vi "OtherDataType.vi"() -> ()   [LabVIEW 2023]
panel:
  out "data":dbl
  out "variant":variant
  in  "Numeric":dbl
  out "Text Ring 2":u16(ring) items=["동", "서", "남", "북"]
  in  "Text Ring":u16(ring) items=["동", "서", "남", "북"]
  out "Array":dbl[](array[numeric])
  out "Sine":dynamicdata(graph)
  out "Waveform Chart":T1(graph)
  in  "stop 3":bool
  out "Waveform Graph 2":dbl[][](graph)
  in  "stop 2":bool
  in  "stop":bool
  out "Waveform Graph":cluster{dbl, dbl, dbl[]}(graph)
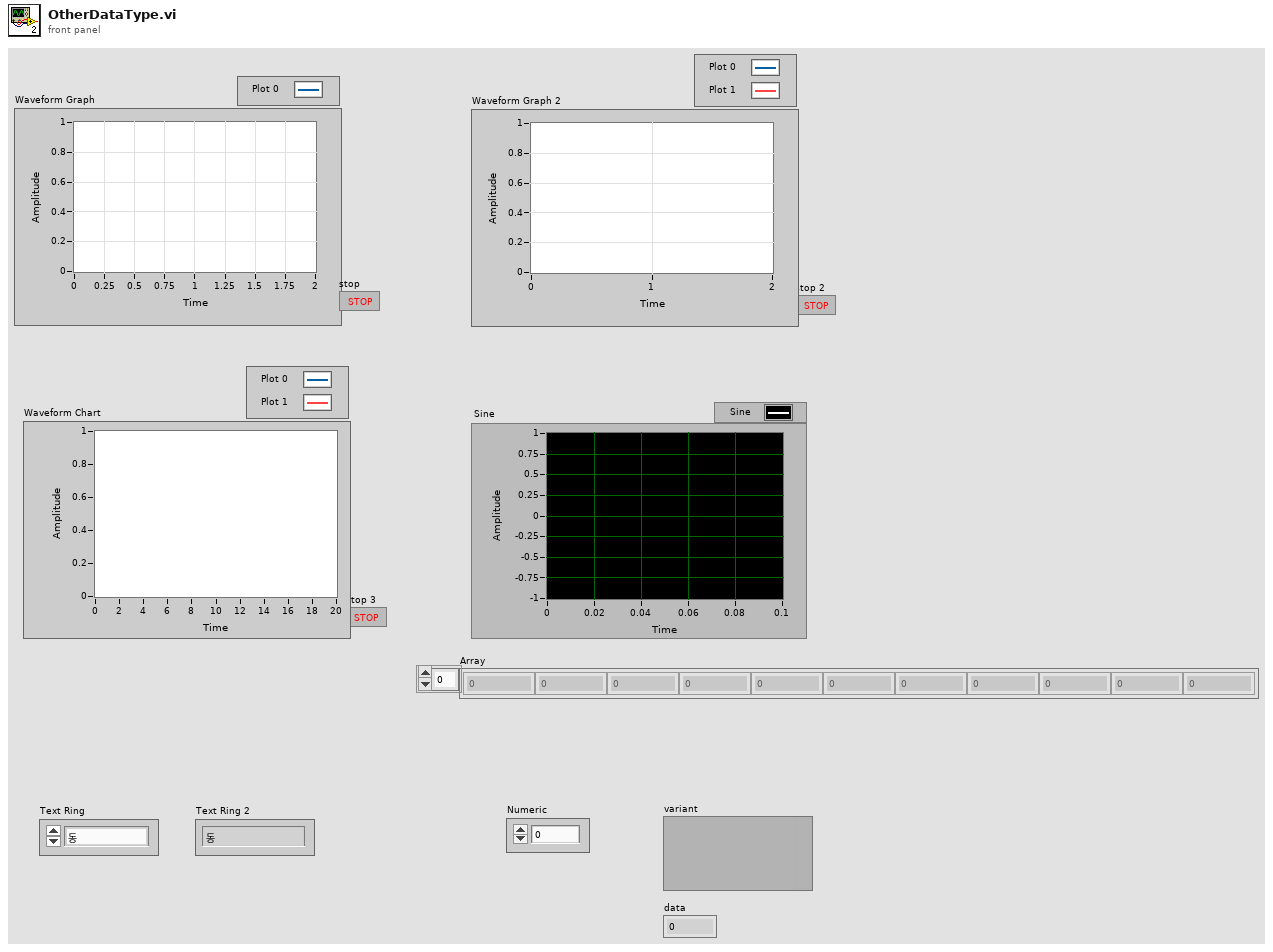
[diagram p1: front panel]
types:
  T1 = cluster{"number: 0 to 1":dbl, "number: 0 to 1":dbl}
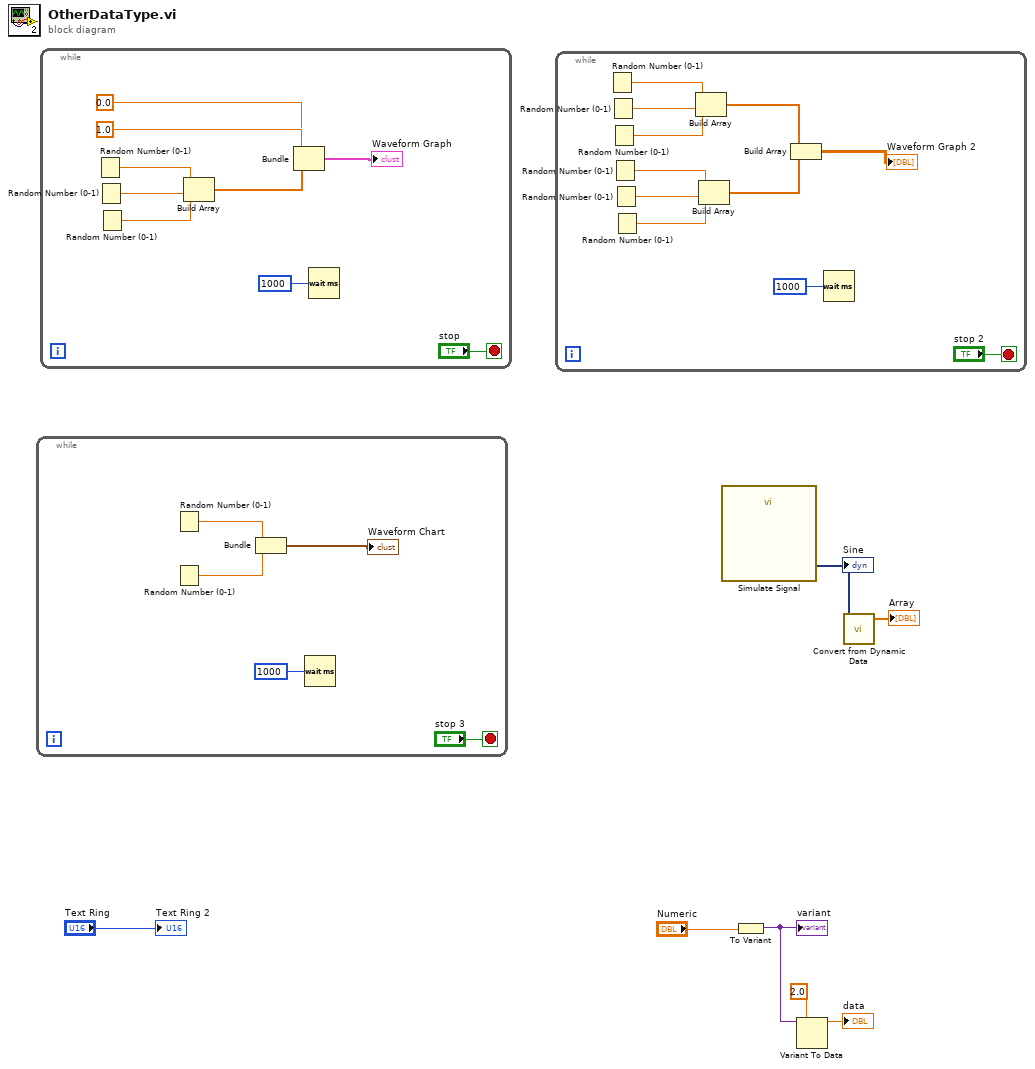
[diagram p0: block diagram]
diagram:
  n1 = while {
    stop <- "stop 3" stop-if-true
    n2 = Random Number (0-1)() -> (number: 0 to 1=w10:dbl)
    n3 = Random Number (0-1)() -> (number: 0 to 1=w9:dbl)
    n4 = Bundle("number: 0 to 1"=w10, "number: 0 to 1"=w9) -> (→"Waveform Chart":T1)  [unwired: 1 in]
    n5 = Wait (ms)(milliseconds to wait=u32 1000) -> ()  [unwired: 1 out]
  }
  n6 = while {
    stop <- "stop" stop-if-true
    n7 = Random Number (0-1)() -> (number: 0 to 1=w21:dbl)
    n8 = Random Number (0-1)() -> (number: 0 to 1=w20:dbl)
    n9 = Random Number (0-1)() -> (number: 0 to 1=w19:dbl)
    n10 = Build Array(w21, w20, w19) -> (w18:dbl[])
    n11 = Bundle(0.0, 1.0, w18) -> (→"Waveform Graph":cluster{dbl, dbl, dbl[]})  [unwired: 1 in]
    n12 = Wait (ms)(milliseconds to wait=u32 1000) -> ()  [unwired: 1 out]
  }
  n13 = while {
    stop <- "stop 2" stop-if-true
    n14 = Random Number (0-1)() -> (number: 0 to 1=w27:dbl)
    n15 = Random Number (0-1)() -> (number: 0 to 1=w26:dbl)
    n16 = Random Number (0-1)() -> (number: 0 to 1=w25:dbl)
    n17 = Random Number (0-1)() -> (number: 0 to 1=w32:dbl)
    n18 = Random Number (0-1)() -> (number: 0 to 1=w31:dbl)
    n19 = Random Number (0-1)() -> (number: 0 to 1=w30:dbl)
    n20 = Build Array(w27, w26, w25) -> (w24:dbl[])
    n21 = Build Array(w32, w31, w30) -> (w23:dbl[])
    n22 = Build Array(w24, w23) -> (→"Waveform Graph 2":dbl[][])
    n23 = Wait (ms)(milliseconds to wait=u32 1000) -> ()  [unwired: 1 out]
  }
  n24 = call "Simulate Signal"() -> ("Sine"=w7:dynamicdata)  [unwired: 14 in, 1 out]
  "Sine" <- w7
  n25 = To Variant(anything="Numeric") -> (Variant=w3:variant)
  "variant" <- w3
  n26 = Variant To Data(type=2.0 ("Numeric"), Variant=w3) -> (data=→"data":dbl)  [unwired: 1 in, 1 out]
  n27 = call "Convert from Dynamic Data"("Dynamic Data Type"=w7) -> ("Array"=→"Array":dbl[])  [unwired: 3 in]
  "Text Ring 2" <- "Text Ring"
